vi "FindUser.vi"(8 "error in (no error)":errorcluster, 11 "被查询者的账号":string) -> (0 "error out":errorcluster, 3 "Array":string[](array[string]))   [LabVIEW 2020]
uses:
  <vilib>/Utility/file.llb/Read Delimited Spreadsheet (string).vi
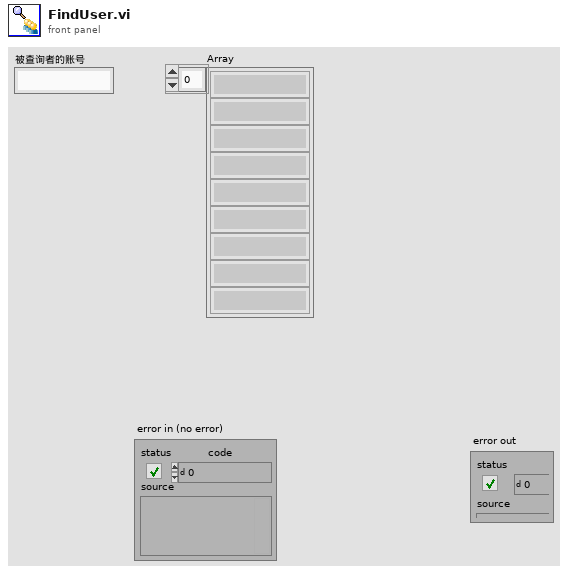
[diagram p1: front panel]
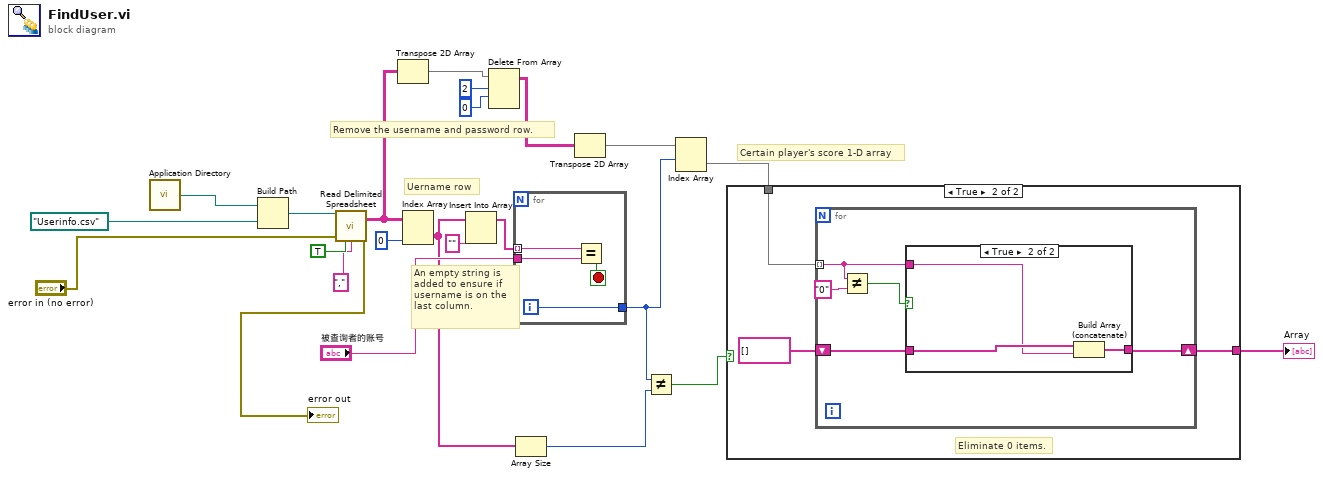
[diagram p0: block diagram]
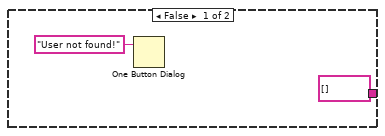
[diagram p2: hidden frame]
diagram:
  # "Certain player's score 1-D array"
  # "Uername row"
  # "An empty string is added to ensure if username is on the last column."
  # "Remove the username and password row."
  n1 = call <vilib>:"Application Directory.vi"() -> ("Application Directory"=w11:path)
  n2 = Build Path(base path=w11, name or relative path=path "Userinfo.csv") -> (appended path=w15:path)
  n3 = call-poly <vilib>:"Read Delimited Spreadsheet.vi"("file path (dialog if empty)"=w15, "error in (no error)"="error in (no error)", "transpose? (F)"=TRUE, "delimiter (\\t)"="," ("delimiter (\\t)")) -> ("all rows"=w19:string[][], "error out"=→"error out":errorcluster)  [unwired: 6 in, 4 out]
  n4 = Transpose 2D Array(2D array=w19) -> (transposed array=w20:string[][])
  n5 = Index Array(array=w19, index (col)=0 ("index (row)")) -> (element=w3:string[])  [unwired: 1 in]
  n6 = Insert Into Array(array=w3, new element="" ("new element/subarray")) -> (w8:string[])  [unwired: 1 in]
  n7 = Delete From Array(array=w20, length=2, index (row)=0) -> (array with subset deleted=w21:string[][])  [unwired: 1 in, 1 out]
  n8 = for {
    tunnel: w8 -> [w27] mode=indexing
    tunnel: "被查询者的账号" -> [w26]
    tunnel: [w24] -> w7
    i -> [w24]
    stop <- w25 stop-if-true
    n9 = Equal?(x=w27, y=w26) -> (x = y?=w25:bool)
  }
  n10 = Array Size(array=w3) -> (size(s)=w6:i32)
  n11 = Transpose 2D Array(2D array=w21) -> (transposed array=w22:string[][])
  n12 = Not Equal?(x=w7, y=w6) -> (x != y?=w5:bool)
  n13 = Index Array(array=w22, index (row)=w7) -> (element=w23:string[])  [unwired: 1 in]
  n14 = case shown="True" w5 {
    tunnel: w23 -> [_ w32]
    tunnel: [string[] [] w30] -> w4
    frame False {
      n15 = One Button Dialog(message="User not found!") -> ()  [unwired: 1 in, 1 out]
    }
    frame True {
      # "Eliminate 0 items."
      n16 = for {
        shift-right: [w36] -> w30
        shift-left: string[] [] -> [w37]
        tunnel: w32 -> [w34] mode=indexing
        n17 = Not Equal?(x=w34, y="0") -> (x != y?=w33:bool)
        n18 = case shown="True" w33 {
          tunnel: w37 -> [w38 w41]
          tunnel: w34 -> [_ w40]
          tunnel: [w38 w39] -> w36
          frame False {
          }
          frame True {
            n19 = Build Array (concatenate)(w41, w40) -> (w39:string[])
          }
        }
      }
    }
  }
  "Array" <- w4
